vi "xcorr.vi"(4 "Delta":u8, 5 "Pulse Energy":fxp<+,32,0>=0.99609375, 6 "N":u8, 7 "y":u32, 8 "x":u32, 9 "enable":bool, 10 "tao":u16) -> (1 "Rxy valid":bool, 2 "Rxy":u64, 3 "trigger":bool)   [LabVIEW 2017]
uses:
  <vilib>/rvi/FXPMathLib/basic elements/FxpDiscreteDelay/XNode/nifxpmath_DiscreteDelay.xnode
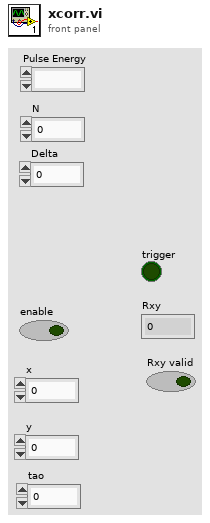
[diagram p1: front panel]
types:
  T1 = cluster{"Q":bool, "Q":bool, "Q":bool, "Q":bool, "Q":bool, "Q":bool, "Q":bool, "Q":bool, "Q":bool, "Q":bool, "Q":bool, "Q":bool, "Q":bool}
  T2 = cluster{"[0]":bool, "[1]":bool, "[2]":bool, "[3]":bool, "[4]":bool, "[5]":bool, "[6]":bool, "[7]":bool, "[8]":bool, "[9]":bool, "[10]":bool, "[11]":bool, "[12]":bool}
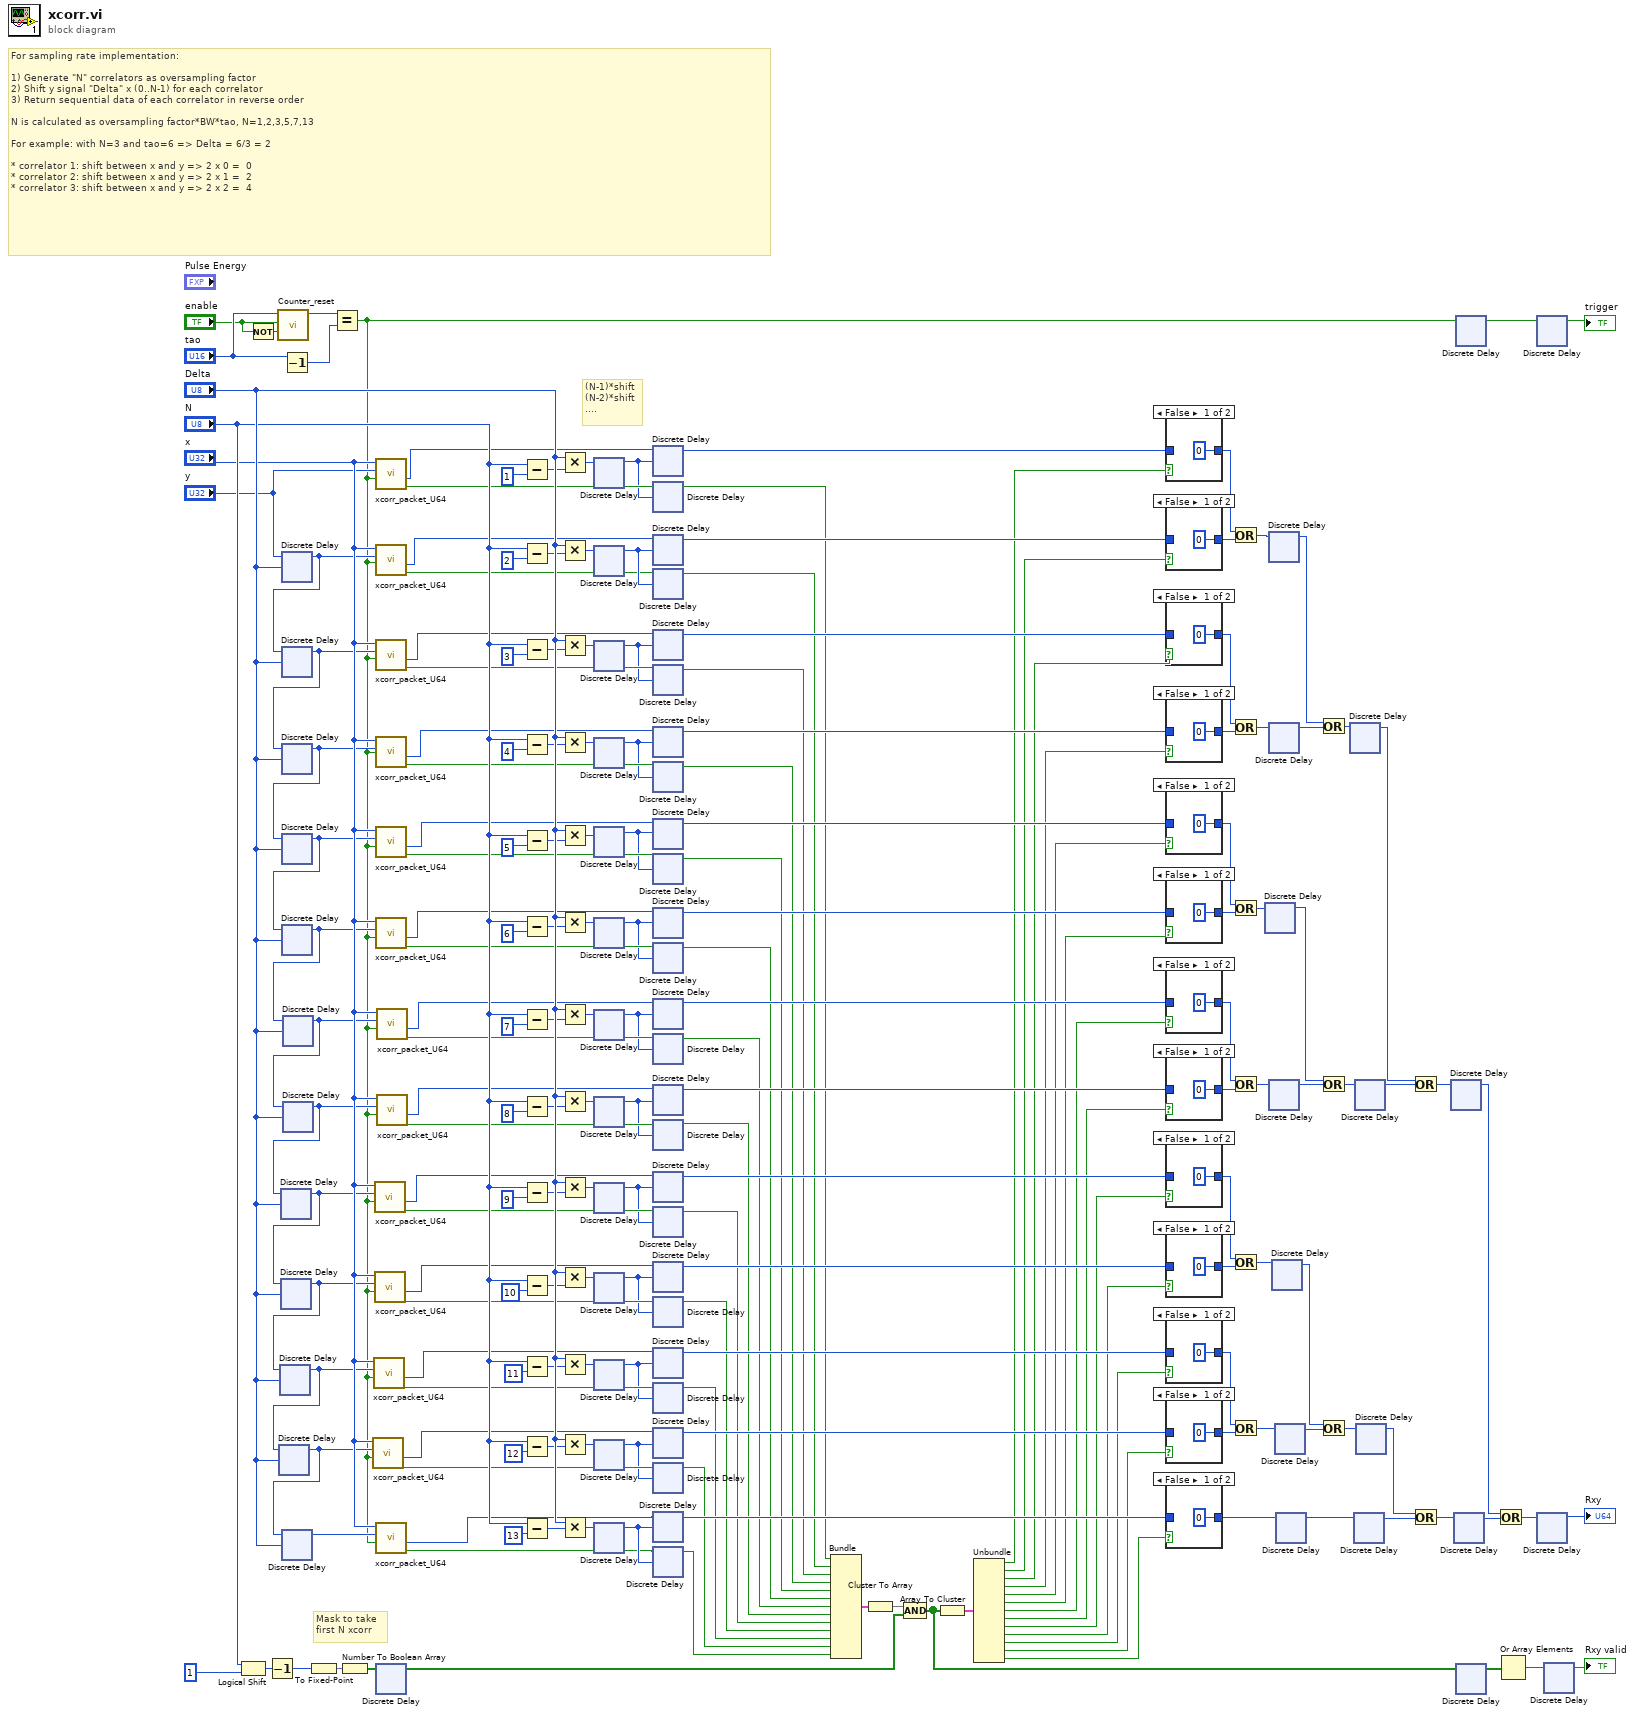
[diagram p0: block diagram]
diagram:
  # "(N-1)*shift\n(N-2)*shift\n...."
  # "Mask to take \nfirst N xcorr"
  # "For sampling rate implementation:\n\n1) Generate \"N\" correlators as oversampling factor\n2) Shift y signal \"Delta\" x (0..N-1) for each correlator\n3) Return sequential data of each correlator in reverse order\n\nN is calculated as oversampling factor*BW*tao, N=1,2,3,5,7,13\n\nFor example: with N=3 and tao=6 => Delta = 6/3 = 2\n\n* correlator 1: shift between x and y => 2 x 0 =  0\n* correlator 2: shift between x and y => 2 x 1 =  2\n* correlator 3: shift between x and y => 2 x 2 =  4"
  n1 = Logical Shift(y="N", x=u16 1) -> (x << y=w186:u16)
  n2 = Not(x="enable") -> (.not. x?=w192:bool)
  n3 = Decrement(x=w186) -> (x-1=w185:u16)
  n4 = call "Counter_reset.vi"("reset"=w192, "enable"="enable", "limit"="tao") -> ("count"=w193:u16)  [unwired: 7 in, 1 out]
  n5 = Decrement(x="tao") -> (x-1=w190:u16)
  n6 = xnode ("Discrete Delay")("D"="y", "n-1[0..255]"="Delta") -> ("Q"=w145:u32)
  n7 = xnode ("Discrete Delay")("D"=w145, "n-1[0..255]"="Delta") -> ("Q"=w155:u32)
  n8 = xnode ("Discrete Delay")("D"=w155, "n-1[0..255]"="Delta") -> ("Q"=w154:u32)
  n9 = xnode ("Discrete Delay")("D"=w154, "n-1[0..255]"="Delta") -> ("Q"=w153:u32)
  n10 = xnode ("Discrete Delay")("D"=w153, "n-1[0..255]"="Delta") -> ("Q"=w152:u32)
  n11 = xnode ("Discrete Delay")("D"=w152, "n-1[0..255]"="Delta") -> ("Q"=w151:u32)
  n12 = xnode ("Discrete Delay")("D"=w151, "n-1[0..255]"="Delta") -> ("Q"=w150:u32)
  n13 = xnode ("Discrete Delay")("D"=w150, "n-1[0..255]"="Delta") -> ("Q"=w149:u32)
  n14 = xnode ("Discrete Delay")("D"=w149, "n-1[0..255]"="Delta") -> ("Q"=w148:u32)
  n15 = xnode ("Discrete Delay")("D"=w148, "n-1[0..255]"="Delta") -> ("Q"=w147:u32)
  n16 = xnode ("Discrete Delay")("D"=w147, "n-1[0..255]"="Delta") -> ("Q"=w146:u32)
  n17 = xnode ("Discrete Delay")("D"=w146, "n-1[0..255]"="Delta") -> ("Q"=w170:u32)
  n18 = To Fixed-Point(number=w185) -> (fixed-point=w184:fxp<+,13,13>)  [unwired: 1 in]
  n19 = Equal?(x=w193, y=w190) -> (x = y?=w2:bool)
  n20 = Number To Boolean Array(number=w184) -> (Boolean array=w182:bool[])
  n21 = call "xcorr_packet_U64.vi"("x"="x", "y"=w146, "trigger"=w2) -> ("out"=w156:u64, "valid"=w159:bool)  [unwired: 5 in]
  n22 = call "xcorr_packet_U64.vi"("x"="x", "y"=w147, "trigger"=w2) -> ("out"=w157:u64, "valid"=w160:bool)  [unwired: 5 in]
  n23 = call "xcorr_packet_U64.vi"("x"="x", "y"=w149, "trigger"=w2) -> ("out"=w163:u64, "valid"=w162:bool)  [unwired: 5 in]
  n24 = call "xcorr_packet_U64.vi"("x"="x", "y"=w148, "trigger"=w2) -> ("out"=w158:u64, "valid"=w161:bool)  [unwired: 5 in]
  n25 = call "xcorr_packet_U64.vi"("x"="x", "y"="y", "trigger"=w2) -> ("out"=w179:u64, "valid"=w178:bool)  [unwired: 5 in]
  n26 = call "xcorr_packet_U64.vi"("x"="x", "y"=w145, "trigger"=w2) -> ("out"=w85:u64, "valid"=w84:bool)  [unwired: 5 in]
  n27 = call "xcorr_packet_U64.vi"("x"="x", "y"=w155, "trigger"=w2) -> ("out"=w175:u64, "valid"=w177:bool)  [unwired: 5 in]
  n28 = call "xcorr_packet_U64.vi"("x"="x", "y"=w154, "trigger"=w2) -> ("out"=w174:u64, "valid"=w176:bool)  [unwired: 5 in]
  n29 = call "xcorr_packet_U64.vi"("x"="x", "y"=w153, "trigger"=w2) -> ("out"=w171:u64, "valid"=w169:bool)  [unwired: 5 in]
  n30 = call "xcorr_packet_U64.vi"("x"="x", "y"=w152, "trigger"=w2) -> ("out"=w172:u64, "valid"=w173:bool)  [unwired: 5 in]
  n31 = call "xcorr_packet_U64.vi"("x"="x", "y"=w170, "trigger"=w2) -> ("out"=w94:u64, "valid"=w93:bool)  [unwired: 5 in]
  n32 = xnode ("Discrete Delay")("D"=w182) -> ("Q"=w91:bool[])
  n33 = call "xcorr_packet_U64.vi"("x"="x", "y"=w151, "trigger"=w2) -> ("out"=w168:u64, "valid"=w167:bool)  [unwired: 5 in]
  n34 = call "xcorr_packet_U64.vi"("x"="x", "y"=w150, "trigger"=w2) -> ("out"=w164:u64, "valid"=w165:bool)  [unwired: 5 in]
  n35 = Subtract(x="N", y=u8 1 ("x")) -> (x-y=w142:u8)
  n36 = Subtract(x="N", y=u8 2 ("x")) -> (x-y=w140:u8)
  n37 = Subtract(x="N", y=u8 3 ("x")) -> (x-y=w138:u8)
  n38 = Subtract(x="N", y=u8 4 ("x")) -> (x-y=w136:u8)
  n39 = Subtract(x="N", y=u8 5 ("x")) -> (x-y=w134:u8)
  n40 = Subtract(x="N", y=u8 6 ("x")) -> (x-y=w132:u8)
  n41 = Subtract(x="N", y=u8 7 ("x")) -> (x-y=w130:u8)
  n42 = Subtract(x="N", y=u8 8 ("x")) -> (x-y=w128:u8)
  n43 = Subtract(x="N", y=u8 9 ("x")) -> (x-y=w126:u8)
  n44 = Subtract(x="N", y=u8 10 ("x")) -> (x-y=w124:u8)
  n45 = Subtract(x="N", y=u8 11 ("x")) -> (x-y=w122:u8)
  n46 = Subtract(x="N", y=u8 12 ("x")) -> (x-y=w121:u8)
  n47 = Subtract(x="N", y=u8 13 ("x")) -> (x-y=w119:u8)
  n48 = Multiply(x="Delta", y=w142) -> (x*y=w86:u8)
  n49 = Multiply(x="Delta", y=w140) -> (x*y=w118:u8)
  n50 = Multiply(x="Delta", y=w138) -> (x*y=w116:u8)
  n51 = Multiply(x="Delta", y=w136) -> (x*y=w114:u8)
  n52 = Multiply(x="Delta", y=w134) -> (x*y=w112:u8)
  n53 = Multiply(x="Delta", y=w132) -> (x*y=w110:u8)
  n54 = Multiply(x="Delta", y=w130) -> (x*y=w108:u8)
  n55 = Multiply(x="Delta", y=w128) -> (x*y=w106:u8)
  n56 = Multiply(x="Delta", y=w126) -> (x*y=w104:u8)
  n57 = Multiply(x="Delta", y=w124) -> (x*y=w102:u8)
  n58 = Multiply(x="Delta", y=w122) -> (x*y=w100:u8)
  n59 = Multiply(x="Delta", y=w121) -> (x*y=w98:u8)
  n60 = Multiply(x="Delta", y=w119) -> (x*y=w96:u8)
  n61 = xnode ("Discrete Delay")("D"=w86) -> ("Q"=w120:u8)
  n62 = xnode ("Discrete Delay")("D"=w118) -> ("Q"=w117:u8)
  n63 = xnode ("Discrete Delay")("D"=w116) -> ("Q"=w115:u8)
  n64 = xnode ("Discrete Delay")("D"=w114) -> ("Q"=w113:u8)
  n65 = xnode ("Discrete Delay")("D"=w112) -> ("Q"=w111:u8)
  n66 = xnode ("Discrete Delay")("D"=w110) -> ("Q"=w109:u8)
  n67 = xnode ("Discrete Delay")("D"=w108) -> ("Q"=w107:u8)
  n68 = xnode ("Discrete Delay")("D"=w106) -> ("Q"=w105:u8)
  n69 = xnode ("Discrete Delay")("D"=w104) -> ("Q"=w103:u8)
  n70 = xnode ("Discrete Delay")("D"=w102) -> ("Q"=w101:u8)
  n71 = xnode ("Discrete Delay")("D"=w100) -> ("Q"=w99:u8)
  n72 = xnode ("Discrete Delay")("D"=w98) -> ("Q"=w97:u8)
  n73 = xnode ("Discrete Delay")("D"=w96) -> ("Q"=w95:u8)
  n74 = xnode ("Discrete Delay")("D"=w179, "n-1[0..255]"=w120) -> ("Q"=w82:u64)
  n75 = xnode ("Discrete Delay")("D"=w178, "n-1[0..255]"=w120) -> ("Q"=w33:bool)
  n76 = xnode ("Discrete Delay")("D"=w85, "n-1[0..255]"=w117) -> ("Q"=w81:u64)
  n77 = xnode ("Discrete Delay")("D"=w84, "n-1[0..255]"=w117) -> ("Q"=w35:bool)
  n78 = xnode ("Discrete Delay")("D"=w175, "n-1[0..255]"=w115) -> ("Q"=w78:u64)
  n79 = xnode ("Discrete Delay")("D"=w177, "n-1[0..255]"=w115) -> ("Q"=w37:bool)
  n80 = xnode ("Discrete Delay")("D"=w174, "n-1[0..255]"=w113) -> ("Q"=w77:u64)
  n81 = xnode ("Discrete Delay")("D"=w176, "n-1[0..255]"=w113) -> ("Q"=w39:bool)
  n82 = xnode ("Discrete Delay")("D"=w171, "n-1[0..255]"=w111) -> ("Q"=w76:u64)
  n83 = xnode ("Discrete Delay")("D"=w169, "n-1[0..255]"=w111) -> ("Q"=w41:bool)
  n84 = xnode ("Discrete Delay")("D"=w172, "n-1[0..255]"=w109) -> ("Q"=w75:u64)
  n85 = xnode ("Discrete Delay")("D"=w173, "n-1[0..255]"=w109) -> ("Q"=w43:bool)
  n86 = xnode ("Discrete Delay")("D"=w168, "n-1[0..255]"=w107) -> ("Q"=w74:u64)
  n87 = xnode ("Discrete Delay")("D"=w167, "n-1[0..255]"=w107) -> ("Q"=w51:bool)
  n88 = xnode ("Discrete Delay")("D"=w164, "n-1[0..255]"=w105) -> ("Q"=w73:u64)
  n89 = xnode ("Discrete Delay")("D"=w165, "n-1[0..255]"=w105) -> ("Q"=w52:bool)
  n90 = xnode ("Discrete Delay")("D"=w163, "n-1[0..255]"=w103) -> ("Q"=w72:u64)
  n91 = xnode ("Discrete Delay")("D"=w162, "n-1[0..255]"=w103) -> ("Q"=w53:bool)
  n92 = xnode ("Discrete Delay")("D"=w158, "n-1[0..255]"=w101) -> ("Q"=w71:u64)
  n93 = xnode ("Discrete Delay")("D"=w161, "n-1[0..255]"=w101) -> ("Q"=w54:bool)
  n94 = xnode ("Discrete Delay")("D"=w157, "n-1[0..255]"=w99) -> ("Q"=w70:u64)
  n95 = xnode ("Discrete Delay")("D"=w160, "n-1[0..255]"=w99) -> ("Q"=w55:bool)
  n96 = xnode ("Discrete Delay")("D"=w156, "n-1[0..255]"=w97) -> ("Q"=w69:u64)
  n97 = xnode ("Discrete Delay")("D"=w159, "n-1[0..255]"=w97) -> ("Q"=w56:bool)
  n98 = xnode ("Discrete Delay")("D"=w94, "n-1[0..255]"=w95) -> ("Q"=w68:u64)
  n99 = xnode ("Discrete Delay")("D"=w93, "n-1[0..255]"=w95) -> ("Q"=w57:bool)
  n100 = Bundle("Q"=w33, "Q"=w35, "Q"=w37, "Q"=w39, "Q"=w41, "Q"=w43, "Q"=w51, "Q"=w52, "Q"=w53, "Q"=w54, "Q"=w55, "Q"=w56, "Q"=w57) -> (w166:T1)  [unwired: 1 in]
  n101 = Cluster To Array(cluster=w166) -> (array=w144:bool[])
  n102 = Compound Arithmetic op=AND(w144, w91) -> (w4:bool[])
  n103 = Array To Cluster(array=w4) -> (cluster=w83:T2)
  n104 = Unbundle(w83) -> ("[0]"=w32:bool, "[1]"=w34:bool, "[2]"=w36:bool, "[3]"=w38:bool, "[4]"=w40:bool, "[5]"=w42:bool, "[6]"=w44:bool, "[7]"=w45:bool, "[8]"=w46:bool, "[9]"=w47:bool, "[10]"=w48:bool, "[11]"=w49:bool, "[12]"=w50:bool)
  n105 = case shown="False" w32 {
    tunnel: w82 -> [_ w195]
    tunnel: [u64 0 ("Q") w195] -> w80
    frame False {
    }
    frame True {
    }
  }
  n106 = case shown="False" w34 {
    tunnel: w81 -> [_ w197]
    tunnel: [u64 0 ("Q") w197] -> w79
    frame False {
    }
    frame True {
    }
  }
  n107 = case shown="False" w36 {
    tunnel: w78 -> [_ w199]
    tunnel: [u64 0 ("Q") w199] -> w66
    frame False {
    }
    frame True {
    }
  }
  n108 = case shown="False" w38 {
    tunnel: w77 -> [_ w201]
    tunnel: [u64 0 ("Q") w201] -> w67
    frame False {
    }
    frame True {
    }
  }
  n109 = case shown="False" w40 {
    tunnel: w76 -> [_ w203]
    tunnel: [u64 0 ("Q") w203] -> w64
    frame False {
    }
    frame True {
    }
  }
  n110 = case shown="False" w42 {
    tunnel: w75 -> [_ w205]
    tunnel: [u64 0 ("Q") w205] -> w65
    frame False {
    }
    frame True {
    }
  }
  n111 = case shown="False" w44 {
    tunnel: w74 -> [_ w207]
    tunnel: [u64 0 ("Q") w207] -> w62
    frame False {
    }
    frame True {
    }
  }
  n112 = case shown="False" w45 {
    tunnel: w73 -> [_ w209]
    tunnel: [u64 0 ("Q") w209] -> w63
    frame False {
    }
    frame True {
    }
  }
  n113 = case shown="False" w46 {
    tunnel: w72 -> [_ w211]
    tunnel: [u64 0 ("Q") w211] -> w60
    frame False {
    }
    frame True {
    }
  }
  n114 = case shown="False" w47 {
    tunnel: w71 -> [_ w213]
    tunnel: [u64 0 ("Q") w213] -> w61
    frame False {
    }
    frame True {
    }
  }
  n115 = case shown="False" w48 {
    tunnel: w70 -> [_ w215]
    tunnel: [u64 0 ("Q") w215] -> w58
    frame False {
    }
    frame True {
    }
  }
  n116 = case shown="False" w49 {
    tunnel: w69 -> [_ w217]
    tunnel: [u64 0 ("Q") w217] -> w59
    frame False {
    }
    frame True {
    }
  }
  n117 = case shown="False" w50 {
    tunnel: w68 -> [_ w219]
    tunnel: [u64 0 ("Q") w219] -> w17
    frame False {
    }
    frame True {
    }
  }
  n118 = Or(x=w80, y=w79) -> (x .or. y?=w29:u64)
  n119 = Or(x=w66, y=w67) -> (x .or. y?=w27:u64)
  n120 = Or(x=w64, y=w65) -> (x .or. y?=w25:u64)
  n121 = Or(x=w62, y=w63) -> (x .or. y?=w23:u64)
  n122 = Or(x=w60, y=w61) -> (x .or. y?=w21:u64)
  n123 = Or(x=w58, y=w59) -> (x .or. y?=w19:u64)
  n124 = xnode ("Discrete Delay")("D"=w25) -> ("Q"=w24:u64)
  n125 = xnode ("Discrete Delay")("D"=w29) -> ("Q"=w28:u64)
  n126 = xnode ("Discrete Delay")("D"=w27) -> ("Q"=w26:u64)
  n127 = xnode ("Discrete Delay")("D"=w23) -> ("Q"=w22:u64)
  n128 = xnode ("Discrete Delay")("D"=w21) -> ("Q"=w20:u64)
  n129 = xnode ("Discrete Delay")("D"=w19) -> ("Q"=w18:u64)
  n130 = xnode ("Discrete Delay")("D"=w17) -> ("Q"=w10:u64)
  n131 = Or(x=w28, y=w26) -> (x .or. y?=w16:u64)
  n132 = Or(x=w24, y=w22) -> (x .or. y?=w14:u64)
  n133 = Or(x=w20, y=w18) -> (x .or. y?=w12:u64)
  n134 = xnode ("Discrete Delay")("D"=w16) -> ("Q"=w15:u64)
  n135 = xnode ("Discrete Delay")("D"=w10) -> ("Q"=w9:u64)
  n136 = xnode ("Discrete Delay")("D"=w14) -> ("Q"=w13:u64)
  n137 = xnode ("Discrete Delay")("D"=w12) -> ("Q"=w11:u64)
  n138 = Or(x=w15, y=w13) -> (x .or. y?=w8:u64)
  n139 = Or(x=w11, y=w9) -> (x .or. y?=w6:u64)
  n140 = xnode ("Discrete Delay")("D"=w8) -> ("Q"=w7:u64)
  n141 = xnode ("Discrete Delay")("D"=w6) -> ("Q"=w5:u64)
  n142 = xnode ("Discrete Delay")("D"=w2) -> ("Q"=w1:bool)
  n143 = xnode ("Discrete Delay")("D"=w4) -> ("Q"=w3:bool[])
  n144 = Or(x=w7, y=w5) -> (x .or. y?=w31:u64)
  n145 = Or Array Elements(Boolean array=w3) -> (logical OR=w89:bool)
  n146 = xnode ("Discrete Delay")("D"=w1) -> ("Q"=→"trigger":bool)
  n147 = xnode ("Discrete Delay")("D"=w31) -> ("Q"=→"Rxy":u64)
  n148 = xnode ("Discrete Delay")("D"=w89) -> ("Q"=→"Rxy valid":bool)
